vi "ExtendedKalmanFilter_SetXHat_Single.vi"(9 "xHat Value":dbl, 10 "Row":i32, 11 "in ExtendedKalmanFiilter":T1) -> (0 "Error":bool, 3 "out ExtendedKalmanFiilter":T1)   [LabVIEW 2019, in "Trajectory_Library.lvlib"]
doc: "Set an element of the initial state estimate x-hat.\n \nInputs:\n - inExtendedKalmanFIlter -- filter data cluster\n - row Row of x-hat.\n - value Value for element of x-hat.\n\nReturns:\n - outExtendedKalmanFIlter -- updated filter data cluster\n - Error -- If TRUE, an error occurred."
uses:
  Trajectory_Library.lvlib
  <vilib>/Analysis/Matrix/Datatypes/RealMatrix.ctl
  <vilib>/Analysis/Matrix/NI_Matrix.lvlib
  TypeDef/EXTENDED_KALMAN_FILTER.ctl
panel:
  # "State Estimate <Statess,1>"
  # "<States, States>"
  # "<States, States>"
  # "<Statess,  States>"
  # "<Outputs, Outputs>"
  # "State Estimate <Statess,1>"
  # "<States, States>"
  # "<States, States>"
  # "<Statess,  States>"
  # "<Outputs, Outputs>"
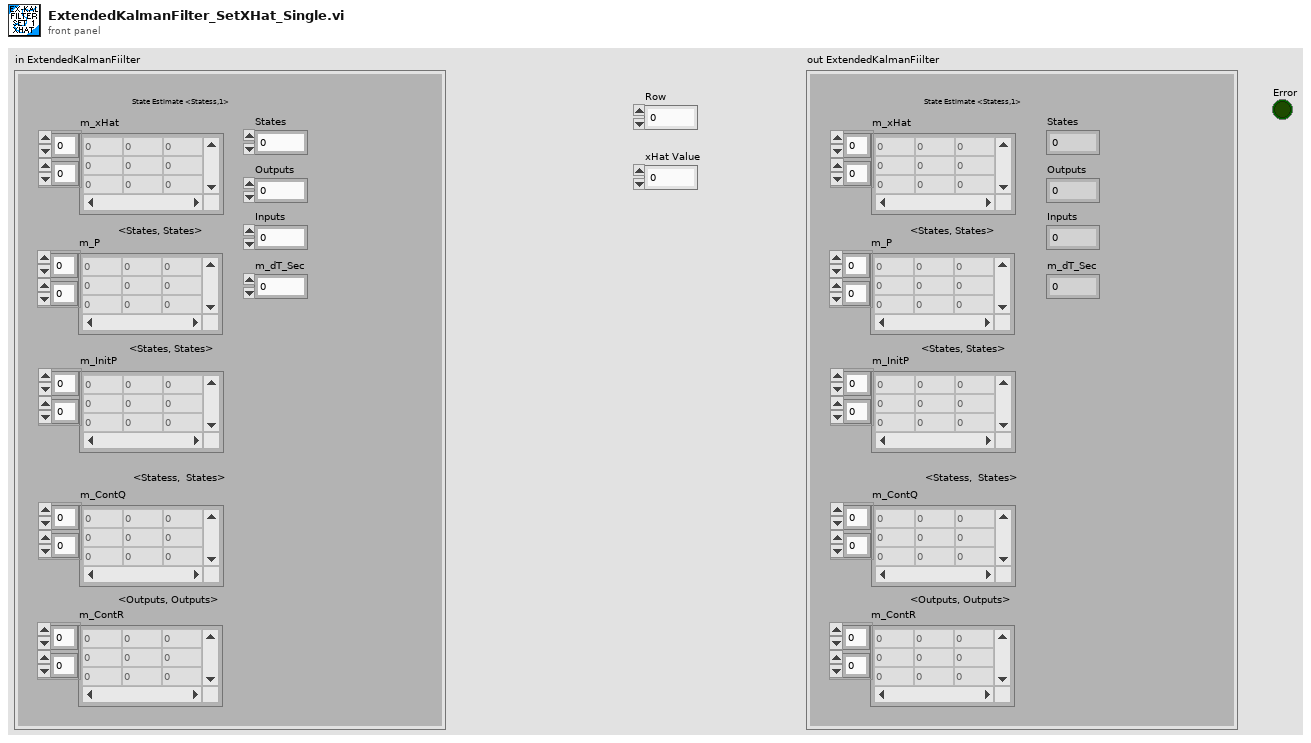
[diagram p1: front panel]
types:
  T1 = typedef "Trajectory_Library.lvlib/EXTENDED_KALMAN_FILTER.ctl" = cluster{"m_P":T2, "m_xHat":T2, "States":i32, "Outputs":i32, "m_ContR":T2, "m_ContQ":T2, "m_dT_Sec":dbl, "Inputs":i32, "m_InitP":T2}
  T2 = typedef "NI_Matrix.lvlib/RealMatrix.ctl" = dbl[][]
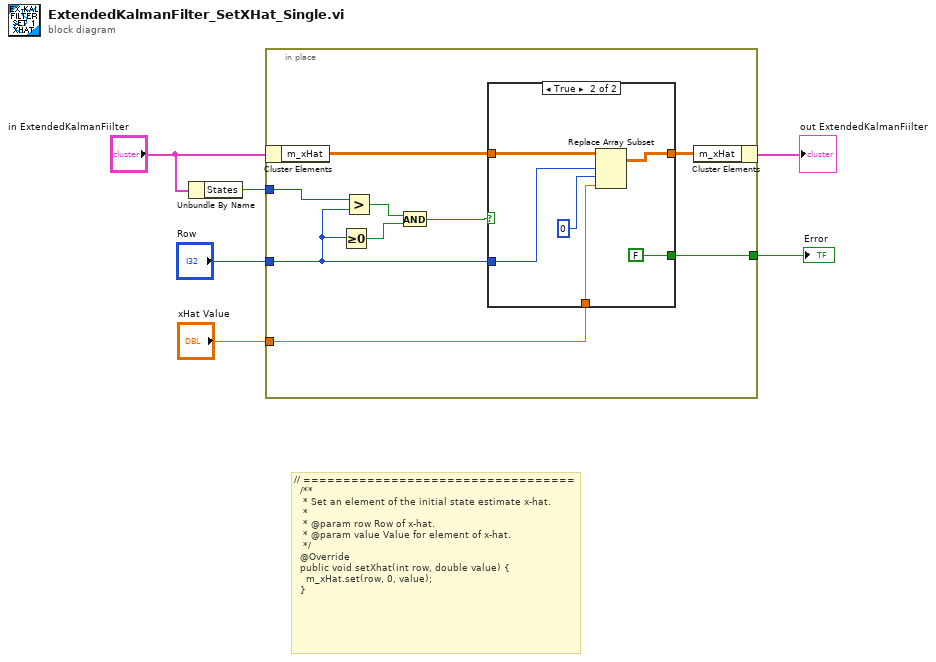
[diagram p0: block diagram]
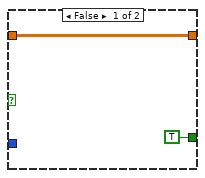
[diagram p2: hidden frame]
diagram:
  # "// ==================================\n  /**\n   * Set an element of the initial state estimate x-hat.\n   *\n   * @param row Row of x-hat.\n   * @param value Value for element of x-hat.\n   */\n  @Override\n  public void setXhat(int row, double value) {\n    m_xHat.set(row, 0, value);\n  }"
  n1 = Unbundle By Name("in ExtendedKalmanFiilter") -> ("States"=w2:i32)
  n2 = in-place {
    in-place-border: "Row" -> [w12]
    in-place-border: "xHat Value" -> [w13]
    in-place-border: w2 -> [w11]
    in-place-border: [w7] -> w1
    n3 = in-place-cluster #1("in ExtendedKalmanFiilter") -> ("m_xHat"=w15:T2)
    n4 = Greater Or Equal To 0?(x=w12) -> (x >= 0?=w9:bool)
    n5 = Greater?(x=w11, y=w12) -> (0:w10:bool)
    n6 = And(x=w10, y=w9) -> (x .and. y?=w8:bool)
    n7 = case shown="True" w8 {
      tunnel: w15 -> [w16 w23]
      tunnel: [w16 w22] -> w14
      tunnel: w12 -> [_ w20]
      tunnel: w13 -> [_ w19]
      tunnel: [TRUE FALSE] -> w7
      frame False {
      }
      frame True {
        n8 = Replace Array Subset(array=w23, new element=w19, index (row)=w20, index (col)=0) -> (w22:T2)
      }
    }
    n9 = in-place-cluster #1("m_xHat"=w14) -> (→"out ExtendedKalmanFiilter":T1)
  }
  "Error" <- w1
